vi "RSZVB Get IMOD Internal Combiner.vi"(8 "error in (no error)":errorcluster {"code" format="%.0x"}, 10 "Channel (1)":i32=1, 11 "VISA session":refnum<visa-resource-name>) -> (0 "error out":errorcluster {"code" format="%.0x"}, 1 "Internal Combiner":bool, 3 "dup VISA session":refnum<visa-resource-name>)   [LabVIEW 2011]
doc: "This VI returns the internal combiner.\n\nNote(s):\n\n(1) This VI requires option R&S ZVT20-B11.\n\nRemote-control command(s):\n[SENSe<Ch>:]FREQuency:IMODulation:COMBiner[:STATe]?"
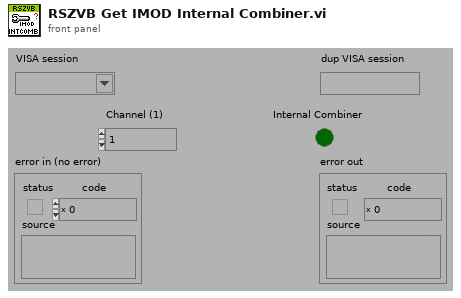
[diagram p1: front panel]
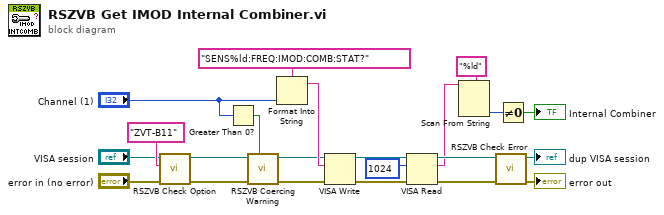
[diagram p0: block diagram]
diagram:
  n1 = call "RSZVB Check Option.vi"("error in (no error)"="error in (no error)", "Options"="ZVT-B11", "VISA session"="VISA session") -> ("error out"=w20:errorcluster, "dup VISA session"=w19:refnum<visa-resource-name>)  [unwired: 7 in]
  n2 = Greater Than 0?(x="Channel (1)") -> (x > 0?=w21:bool)
  n3 = call "RSZVB Coercing Warning.vi"("In Range?"=w21, "error in (no error)"=w20, "VISA session"=w19) -> ("error out"=w18:errorcluster, "dup VISA session"=w17:refnum<visa-resource-name>)  [unwired: 7 in]
  n4 = Format Into String(format string="SENS%ld:FREQ:IMOD:COMB:STAT?", "Channel (1)") -> (resulting string=w22:string)  [unwired: 2 in, 1 out]
  n5 = VISA Write(VISA resource name=w17, write buffer=w22, error in (no error)=w18) -> (VISA resource name out=w8:refnum<visa-resource-name>, error out=w7:errorcluster)  [unwired: 1 out]
  n6 = VISA Read(VISA resource name=w8, byte count=u32 1024 ("byte count (0)"), error in (no error)=w7) -> (VISA resource name out=w6:refnum<visa-resource-name>, read buffer=w1:string, error out=w5:errorcluster)  [unwired: 1 out]
  n7 = Scan From String(format string="%ld", input string=w1) -> (output 1=w3:i32)  [unwired: 3 in, 3 out]
  n8 = call "RSZVB Check Error.vi"("error in (no error)"=w5, "VISA session"=w6) -> ("error out"=→"error out":errorcluster, "dup VISA session"=→"dup VISA session":refnum<visa-resource-name>)  [unwired: 8 in]
  n9 = Not Equal To 0?(x=w3) -> (x != 0?=→"Internal Combiner":bool)
